vi "Set - Wash Steps.vi"(8 "error in (no error)":errorcluster, 9 "Next Wash Step":T1, 10 "Current Wash Step":T1, 11 "View Model":T2) -> (0 "error out":errorcluster, 3 "View Model":T2)   [LabVIEW 2017]
doc: "Get actual value of Wash Steps from DVR."
uses:
  Controls/View Model.ctl
  Controls/Shared Model.ctl
  Error Handler/Controls/Error Model.ctl
  Error Handler/Controls/Error Data.ctl
  Error Handler/Controls/Error Level.ctl
  Configuration/Controls/Config Model.ctl
  Configuration/Controls/Config Record.ctl
  Configuration/Controls/Config Data.ctl
  Configuration/Controls/Config Command.ctl
  Controller/Controls/Controler Model.ctl
  Views/Entry Console View/Controls/Entry Console - Wash Steps.ctl
  Controller/Controls/Controller - Overhead.ctl
  Controller/Controls/Controller - States.ctl
  Controller/Controls/Controller - Wash Step.ctl
  Views/Vehicle Position View/Controls/Vehicle - Station Enum.ctl
  Controller/Controls/Controller - Event.ctl
  Controller/Controls/Controller - Commands.ctl
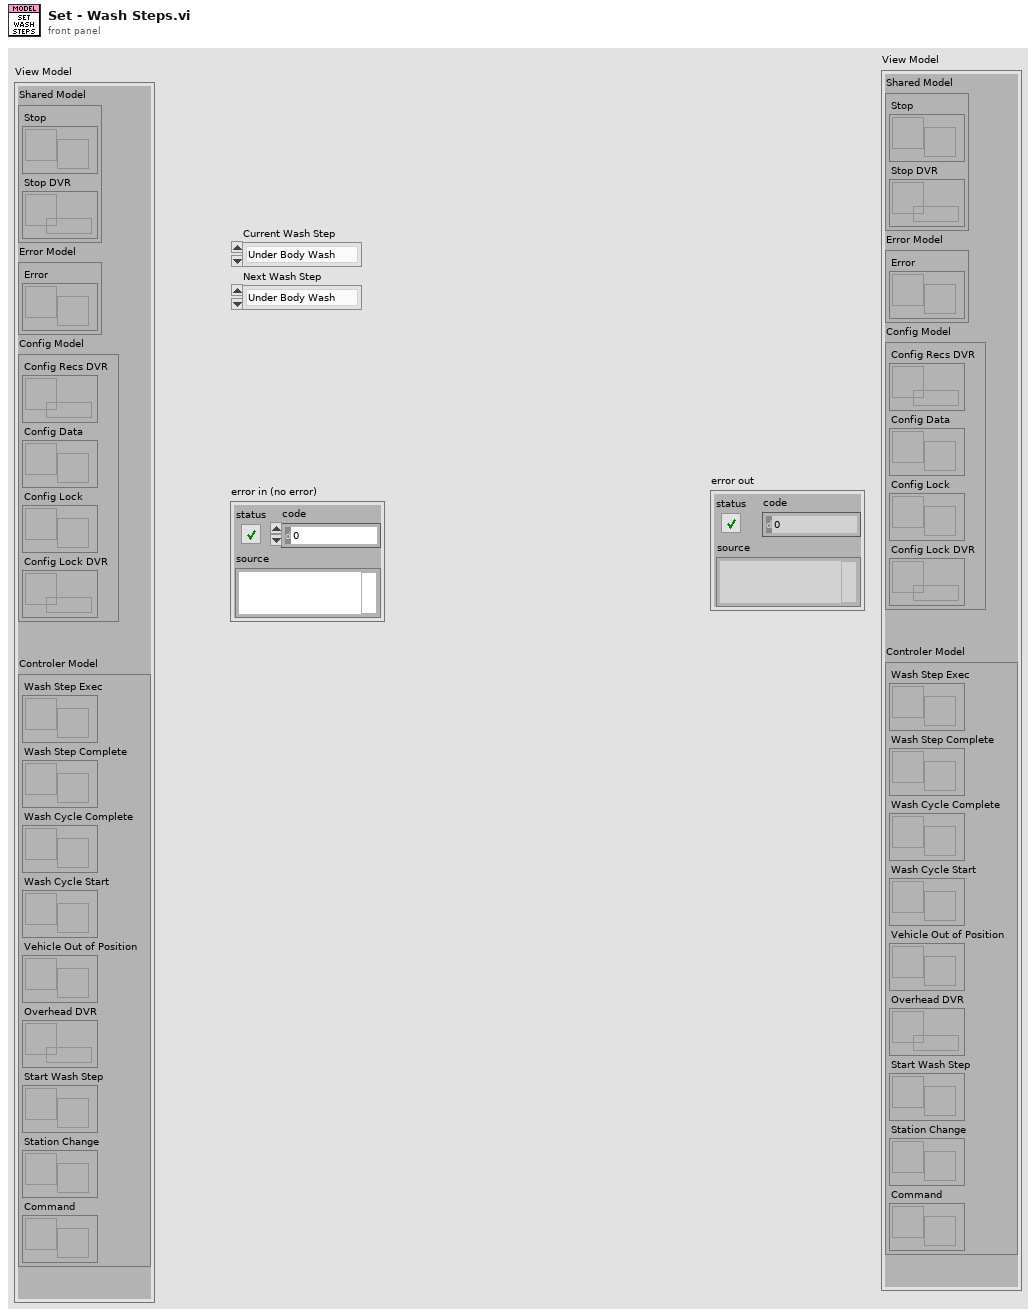
[diagram p1: front panel]
types:
  T1 = typedef "Controller - Wash Step.ctl" = enum16{"Under Body Wash", "Bug Remover", "Pre-Soak", "High Pressure Wash", "Low Pressure Wax", "Spot Free Rinse", "Tire Shine Foam", "Air Dry"}
  T2 = typedef "View Model.ctl" = cluster{"Shared Model":T3, "Error Model":T4, "Config Model":T5, "Controler Model":T6}
  T3 = typedef "Shared Model.ctl" = cluster{"Stop":refnum<user-event>, "Stop DVR":refnum<data-value>}
  T4 = typedef "Error Model.ctl" = cluster{"Error":refnum<user-event>}
  T5 = typedef "Config Model.ctl" = cluster{"Config Recs DVR":refnum<data-value>, "Config Data":refnum<user-event>, "Config Lock":refnum<user-event>, "Config Lock DVR":refnum<data-value>}
  T6 = typedef "Controler Model.ctl" = cluster{"Wash Step Exec":refnum<user-event>, "Wash Step Complete":refnum<user-event>, "Wash Cycle Complete":refnum<user-event>, "Wash Cycle Start":refnum<user-event>, "Vehicle Out of Position":refnum<user-event>, "Overhead DVR":refnum<data-value>, "Start Wash Step":refnum<user-event>, "Station Change":refnum<user-event>, "Command":refnum<user-event>}
  T7 = typedef "Controller - Overhead.ctl" = cluster{"Vehicle on Position?":bool, "Step Duration":u32, "Elapsed Time":dbl, "State":T8, "Next State":T8, "Current Wash Step":T1, "Next Wash Step":T1, "Wash Sequence":T1[], "Current Station":T9}
  T8 = typedef "Controller - States.ctl" = enum16{"Initial", "Wait for Start", "Wash Cycle Start", "Wait for Vehicle Position", "Wash Step Start", "Wash Step Execute", "Wash Step Complete", "Wash Cycle Complete", "Wash Exit", "Wash Abort/Terminate"}
  T9 = typedef "Vehicle - Station Enum.ctl" = enum16{"Entry", "Station1", "Station2", "Station3", "Exit"}
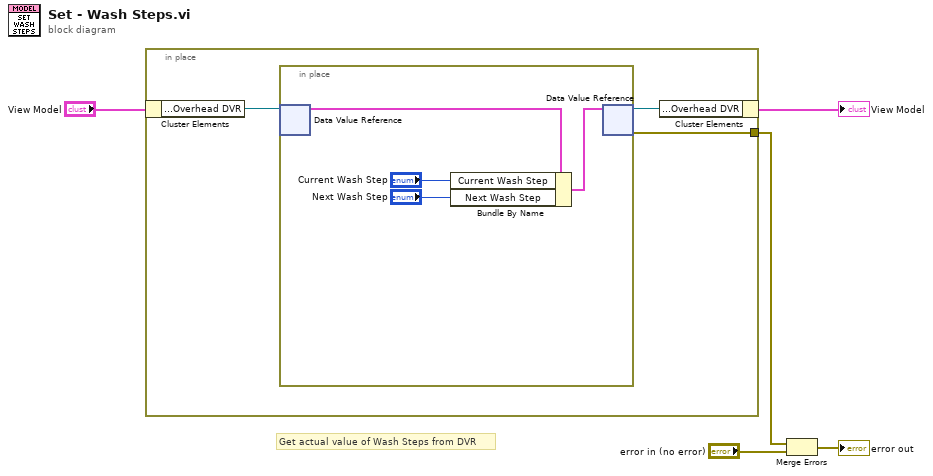
[diagram p0: block diagram]
diagram:
  # "Get actual value of Wash Steps from DVR"
  n1 = in-place {
    in-place-border: [w6] -> w2
    n2 = in-place-cluster #1("View Model") -> ("Controler Model.Overhead DVR"=w8:refnum<data-value>)
    n3 = in-place {
      n4 = in-place-dvr #2(w8) -> (w12:T7)  [unwired: 1 out]
      n5 = Bundle By Name(cluster=w12, "Current Wash Step"="Current Wash Step", "Next Wash Step"="Next Wash Step") -> (w11:T7)
      n6 = in-place-dvr #2(w11) -> (w7:refnum<data-value>, w6:errorcluster)
    }
    n7 = in-place-cluster #1("Controler Model.Overhead DVR"=w7) -> (→"View Model":T2)
  }
  n8 = Merge Errors(w2, "error in (no error)") -> (→"error out":errorcluster)
